vi "Run_Sub Function.vi"(0 "functionbase in":refnum<class "functionbase.lvclass">, 5 "Sub Function":T1[](array[typedef]), 11 "error in (no error)":errorcluster) -> (4 "functionbase out":refnum<class "functionbase.lvclass">, 15 "error out":errorcluster)   [LabVIEW 2016, in "functionbase.lvclass"]
uses:
  functionbase.lvclass
  common/line and indent/Function Indent Combo.ctl
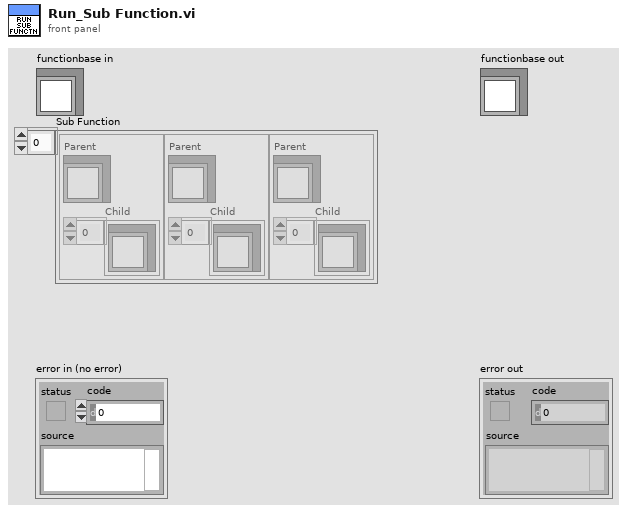
[diagram p1: front panel]
types:
  T1 = typedef "Function Indent Combo.ctl" = cluster{"Parent":refnum<class "functionbase.lvclass">, "Child":refnum<class "functionbase.lvclass">[]}
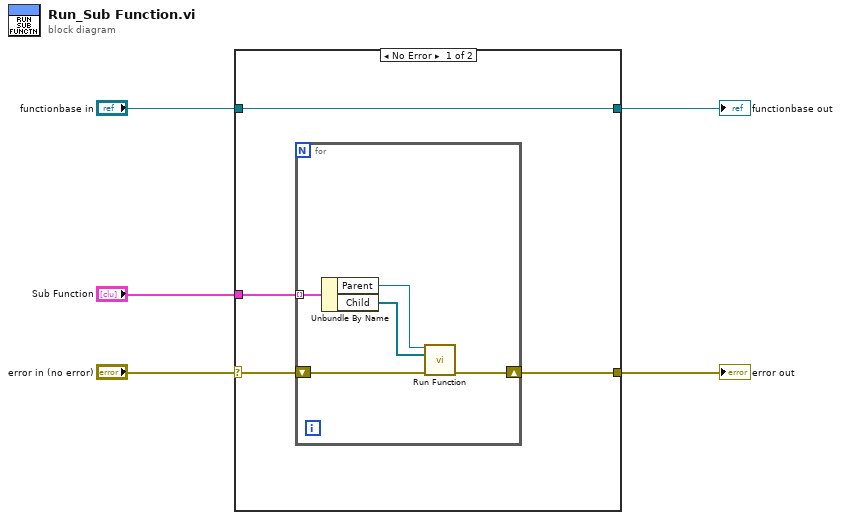
[diagram p0: block diagram]
diagram:
  n1 = case shown="No Error" "error in (no error)" {
    selector: "error in (no error)" -> [w8 w16]
    tunnel: [w7 w16] -> w4
    tunnel: [w9 w15] -> w2
    tunnel: "functionbase in" -> [w9 w15]
    tunnel: "Sub Function" -> [w6 _]
    frame No Error {
      n2 = for {
        tunnel: w6 -> [w14] mode=indexing
        shift-right: [w11] -> w7
        shift-left: w8 -> [w12]
        n3 = Unbundle By Name(w14) -> ("Parent"=w13:refnum<class "functionbase.lvclass">, "Child"=w10:refnum<class "functionbase.lvclass">[])
        n4 = call-dynamic "Run Function.vi"("functionbase in"=w13, "Sub Functions"=w10, "error in (no error)"=w12) -> ("error out"=w11:errorcluster)  [unwired: 10 in, 2 out]
      }
    }
    frame Error {
    }
  }
  "error out" <- w4
  "functionbase out" <- w2
